vi "main.vi"(8 "stop":bool) -> (0 "sensor_value":u32, 3 "who am I ?":bool[](array[boolean]))   [LabVIEW 2019]
uses:
  <vilib>/rvi/Emulation/niFpgaGetClockAttributes.vi
  <vilib>/rvi/Emulation/niFpgaSctlEmulationGetInTimedLoop.vi
  <vilib>/rvi/Emulation/niFpgaEmulationReportErrorSimple.vi
  <vilib>/rvi/Emulation/niFpgaCriticalErrorInLSC.vi
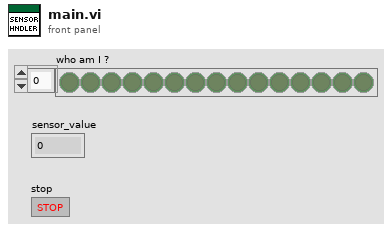
[diagram p1: front panel]
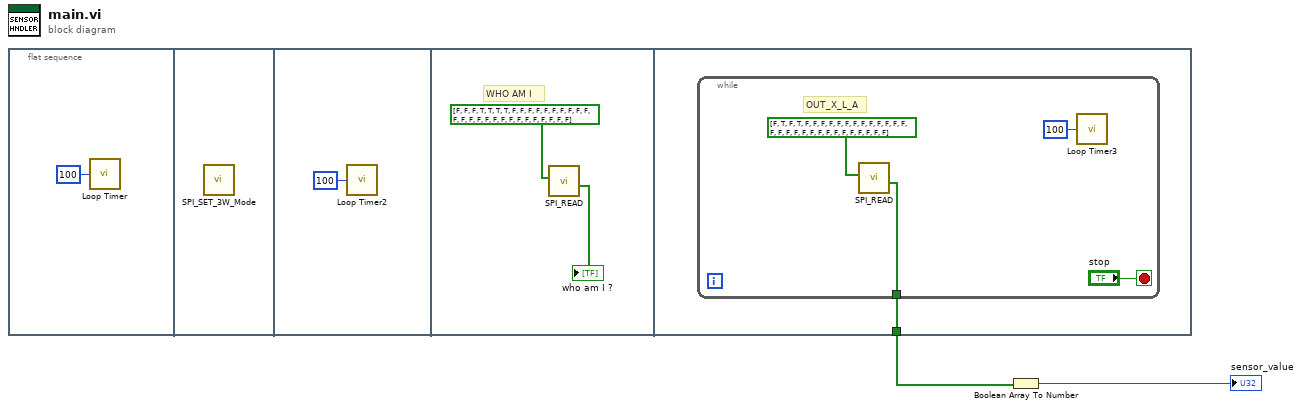
[diagram p0: block diagram]
diagram:
  n1 = flat-sequence {
    tunnel: [w7] -> w2
    frame #0 {
      n2 = call "Loop Timer"("Count(mSec)"=u32 100 ("Count(Ticks)")) -> ()  [unwired: 1 out]
    }
    frame #1 {
      n3 = call "SPI_SET_3W_Mode.vi"() -> ()  [unwired: 12 in]
    }
    frame #2 {
      n4 = call "Loop Timer2"("Count(mSec)"=u32 100 ("Count(Ticks)")) -> ()  [unwired: 1 out]
    }
    frame #3 {
      # "WHO AM I"
      n5 = call "SPI_READ.vi"("Register_adress"=bool[] [FALSE, FALSE, FALSE, TRUE, TRUE, TRUE, TRUE, FALSE, FALSE, FALSE, FALSE, FALSE, FALSE, FALSE, FALSE, FALSE, FALSE, FALSE, FALSE, FALSE, FALSE, FALSE, FALSE, FALSE, FALSE, FALSE, FALSE, FALSE, FALSE, FALSE, FALSE, FALSE]) -> ("msg"=→"who am I ?":bool[])  [unwired: 9 in]
    }
    frame #4 {
      n6 = while {
        tunnel: [w8] -> w7
        stop <- "stop" stop-if-true
        # "OUT_X_L_A"
        n7 = call "SPI_READ.vi"("Register_adress"=bool[] [FALSE, TRUE, FALSE, TRUE, FALSE, FALSE, FALSE, FALSE, FALSE, FALSE, FALSE, FALSE, FALSE, FALSE, FALSE, FALSE, FALSE, FALSE, FALSE, FALSE, FALSE, FALSE, FALSE, FALSE, FALSE, FALSE, FALSE, FALSE, FALSE, FALSE, FALSE, FALSE]) -> ("msg"=w8:bool[])  [unwired: 9 in]
        n8 = call "Loop Timer3"("Count(mSec)"=u32 100 ("Count(Ticks)")) -> ()  [unwired: 1 out]
      }
    }
  }
  n9 = Boolean Array To Number(Boolean array=w2) -> (number=→"sensor_value":u32)
